vi "Robot Global Data.vi"() -> ()   [LabVIEW 2013]
doc: "This global VI can contain as many global variables as you need. Place a control on the panel, give it a good name. To read or write to it from a VI, drag the icon to the diagram of that VI. You can also drag from the project. Click on the node to change which global you access. You shouldn't have multiple locations writing to a global or it will cause a race-condition."
uses:
  <vilib>/Rock Robotics/WPI/Camera/WPI_CameraImageSize.ctl
  <vilib>/Rock Robotics/WPI/DriverStation/WPI_DriverStationRobotMode2.ctl
  <vilib>/Rock Robotics/WPI/Relay/WPI_RelayValue.ctl
  Shooter state.ctl
panel:
  in  "Cheesy Vision":T1
  in  "High gear enabled":bool=TRUE
  in  "teleop arm and shoot state":T2
  in  "Target Found":bool
  in  "Compressor":T3=enum."Forward"
  in  "Robot Mode":T4
  in  "LED toggle rate (ms)":u32=20
  in  "image size":T5=enum."320x240"
  in  "Enable Vision":bool
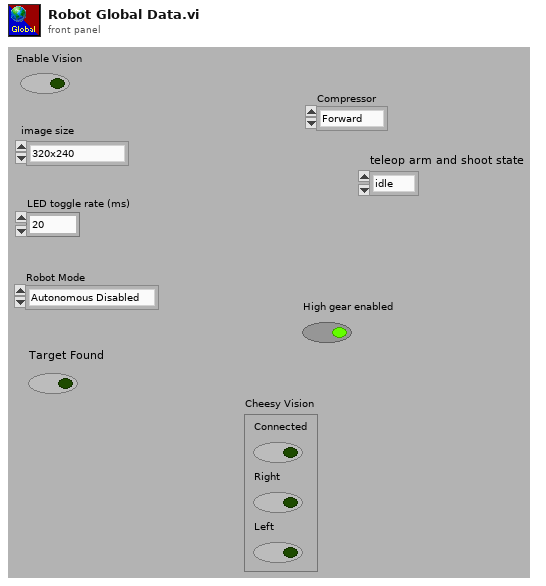
[diagram p1: front panel]
types:
  T1 = cluster{"Connected":bool, "Right":bool, "Left":bool}
  T2 = typedef "Shooter state.ctl" = enum16{"idle", "shoot", "pass", "grab out", "grab in", "reset", "catch", "truss"}
  T3 = typedef "WPI_RelayValue.ctl" = enum16{"Off", "On", "Forward", "Reverse"}
  T4 = typedef "WPI_DriverStationRobotMode2.ctl" = enum16{"Autonomous Disabled", "Autonomous Enabled", "Teleop Disabled", "Teleop Enabled", "Timeout", "Finish", "Test Disabled", "Test Enabled"}
  T5 = typedef "WPI_CameraImageSize.ctl" = enum16{"640x480", "320x240", "160x120"}
diagram:
